vi "send message.vi"(8 "error in (no error)":errorcluster, 11 "Socket in":refnum<class "Socket2.lvclass">) -> (0 "error out":errorcluster, 3 "Socket out":refnum<class "Socket2.lvclass">)   [LabVIEW 2018, in "Socket2.lvclass"]
uses:
  Socket2.lvclass
  Socket2.lvclass/Socket2.ctl
  <vilib>/addons/zeromq/zmq_socket.lvclass
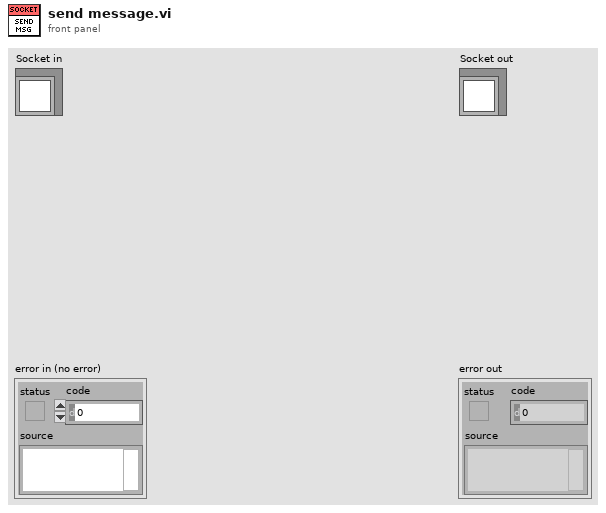
[diagram p1: front panel]
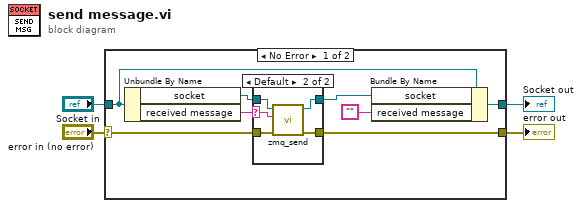
[diagram p0: block diagram]
diagram:
  n1 = case shown="No Error" "error in (no error)" {
    selector: "error in (no error)" -> [w12 w21]
    tunnel: [w11 w21] -> w3
    tunnel: [w8 w20] -> w1
    tunnel: "Socket in" -> [w9 w20]
    frame No Error {
      n2 = Unbundle By Name(w9) -> ("socket"=w10:refnum<class "zmq_socket.lvclass">, "received message"=w6:string)
      n3 = case shown="Default" w6 {
        selector: w6 -> [_ w15]
        tunnel: w12 -> [w13 w19]
        tunnel: [w13 w18] -> w11
        tunnel: w10 -> [w14 w17]
        tunnel: [w14 w16] -> w7
        frame "" {
        }
        frame Default {
          n4 = call <vilib>:"zmq_send.vi"("error in"=w19, "data"=w15, "socket in"=w17) -> ("error out"=w18:errorcluster, "socket out"=w16:refnum<class "zmq_socket.lvclass">)  [unwired: 4 in]
        }
      }
      n5 = Bundle By Name(cluster=w9, "socket"=w7, "received message"="") -> (w8:refnum<class "Socket2.lvclass">)
    }
    frame Error {
    }
  }
  "error out" <- w3
  "Socket out" <- w1
